vi "ProdaNG.TestStep.Set.vi"(8 "error in (no error)":errorcluster, 9 "ReleaseId":T1=enum."released", 10 "TestStep":T2, 11 "dbHandleIn":i32) -> (0 "error out":errorcluster, 2 "TestStep out":T2, 3 "dbHandle":i32)   [LabVIEW 2016]
doc: "This function returns a product structure for a product, which is identified by a part and a serial number.\nImportant information: The field 'individual' was taken over from the field 'allgemein' of the legacy data directly. Because of this most products have the value 0 further on and only a few the value 1. \nParameter:\nhandle is an Integer, which is returned by the function Login() at the creation of a new connection.\nwabcoPartId is the Id of the part.\nserialNumber is the serial number of the product for the part above.\nproduct is a pointer on a product structure, which is filled if the returncode is 0. The structure must be defined in the calling program.\n\nReturncodes:\n0 No error\n< 0 ORACLE Error code\n6 (ERROR_INVALID_HANDLE) in case of an invalid handle\n1403 Record does not exist"
uses:
  Controls/ProdaNG.TestStep.ctl
  Controls/ProdaNG.ReleaseId.ctl
  Controls/ProdaNG.TestStepSize.ctl
  prodllNG.dll
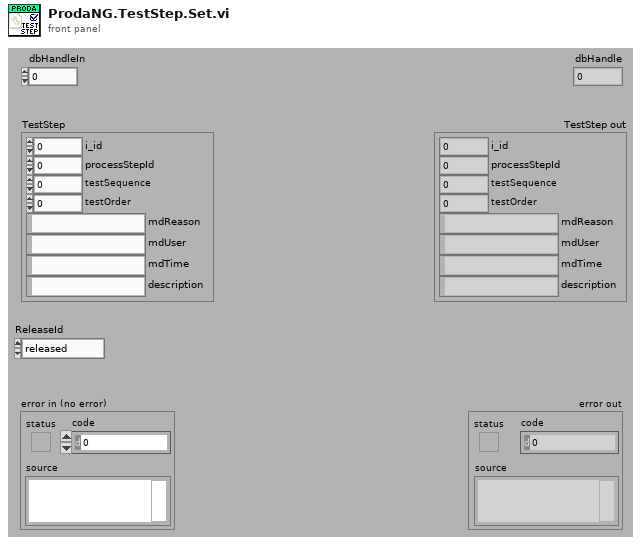
[diagram p1: front panel]
types:
  T1 = typedef "ProdaNG.ReleaseId.ctl" = enum16{"not released", "released", "was released"}
  T2 = typedef "ProdaNG.TestStep.ctl" = cluster{"i_id":i32, "processStepId":i32, "testSequence":i32, "testOrder":i32, "mdReason":string, "mdUser":string, "mdTime":string, "description":string}
  T3 = typedef "ProdaNG.TestStepSize.ctl" = cluster{"i_id":i32, "processStepId":i32, "testSequence":i32, "testOrder":i32, "mdReason":i32, "mdUser":i32, "mdTime":i32, "description":i32}
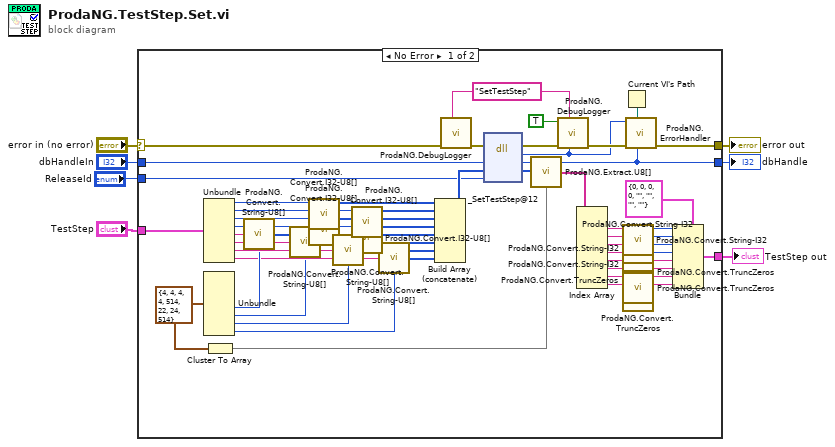
[diagram p0: block diagram]
diagram:
  n1 = case shown="No Error" "error in (no error)" {
    selector: "error in (no error)" -> [w58 w65]
    tunnel: [w63 w65] -> w6
    tunnel: "dbHandleIn" -> [w60 w64]
    tunnel: [w61 w64] -> w4
    tunnel: "TestStep" -> [w24 _]
    tunnel: [w9 _] -> w2
    tunnel: "ReleaseId" -> [w8 _]
    frame No Error {
      w25 = T3 {"i_id"=4, "processStepId"=4, "testSequence"=4, "testOrder"=4, "mdReason"=514, "mdUser"=22, "mdTime"=24, "description"=514} ("TestStepSize")
      w54 = "SetTestStep" ("cmd")
      n2 = Unbundle(w24) -> ("i_id"=w50:i32, "processStepId"=w51:i32, "testSequence"=w20:i32, "testOrder"=w19:i32, "mdReason"=w48:string, "mdUser"=w16:string, "mdTime"=w46:string, "description"=w15:string)
      n3 = Unbundle(w25) -> ("mdReason"=w44:i32, "mdUser"=w12:i32, "mdTime"=w43:i32, "description"=w13:i32)  [unwired: 4 out]
      n4 = Cluster To Array(cluster=w25) -> (array=w21:i32[])
      n5 = call "ProdaNG.Convert.String-U8[].vi"("Input String"=w48, "Size"=w44) -> ("Output"=w47:u8[])
      n6 = call "ProdaNG.Convert.String-U8[].vi"("Input String"=w16, "Size"=w12) -> ("Output"=w10:u8[])
      n7 = call "ProdaNG.Convert.I32-U8[].vi"("32bit integer"=w50) -> ("unsigned byte array"=w49:u8[])  [unwired: 10 in]
      n8 = call "ProdaNG.Convert.I32-U8[].vi"("32bit integer"=w20) -> ("unsigned byte array"=w17:u8[])  [unwired: 10 in]
      n9 = call "ProdaNG.Convert.String-U8[].vi"("Input String"=w46, "Size"=w43) -> ("Output"=w45:u8[])
      n10 = call "ProdaNG.Convert.I32-U8[].vi"("32bit integer"=w51) -> ("unsigned byte array"=w52:u8[])  [unwired: 10 in]
      n11 = call "ProdaNG.Convert.I32-U8[].vi"("32bit integer"=w19) -> ("unsigned byte array"=w18:u8[])  [unwired: 10 in]
      n12 = call "ProdaNG.Convert.String-U8[].vi"("Input String"=w15, "Size"=w13) -> ("Output"=w14:u8[])
      n13 = Build Array (concatenate)(w49, w52, w17, w18, w47, w10, w45, w14) -> (w23:u8[])
      n14 = call "ProdaNG.DebugLogger.vi"("cmd"=w54, "error in (no error)"=w58) -> ("error out"=w57:errorcluster)  [unwired: 9 in]
      n15 = dll-call lib="D:/Maszup/WABCO/SVN/LineTraceSystem/SOFTWARE/sources/Database/ProdaNG/prodllNG.dll" fn="_SetTestStep@12" ("ProDLL wrapper.dll:ProDLL_wrapper_GetWabcoParts_GetData")(error in=w57, "dbHandle"=w60, "testStep"=w23, "releaseId"=w8) -> (error out=w56:errorcluster, "return type"=w53:i32, "dbHandle"=w61:i32, "testStep"=w22:u8[])  [unwired: 3 in, 1 out]
      n16 = call "ProdaNG.Extract.U8[].vi"("unsigned byte array"=w22, "Sizes"=w21) -> ("Elements"=w42:string[])
      n17 = call "ProdaNG.DebugLogger.vi"("return type"=w53, "cmd"=w54, "error in (no error)"=w56, "done? (F)"=TRUE) -> ("error out"=w55:errorcluster)  [unwired: 7 in]
      n18 = Index Array(array=w42) -> (element #1=w41:string, element #2=w38:string, element #3=w37:string, element #4=w31:string, element #5=w28:string, element #6=w27:string, element #7=w32:string, element #8=w34:string)  [unwired: 8 in]
      n19 = Current VI's Path() -> (path=w62:path)
      n20 = call "ProdaNG.Convert.String-I32.vi"("unsigned byte string"=w41) -> ("32bit integer"=w40:i32)  [unwired: 10 in]
      n21 = call "ProdaNG.Convert.String-I32.vi"("unsigned byte string"=w38) -> ("32bit integer"=w39:i32)  [unwired: 10 in]
      n22 = call "ProdaNG.Convert.String-I32.vi"("unsigned byte string"=w37) -> ("32bit integer"=w36:i32)  [unwired: 10 in]
      n23 = call "ProdaNG.Convert.String-I32.vi"("unsigned byte string"=w31) -> ("32bit integer"=w30:i32)  [unwired: 10 in]
      n24 = call "ProdaNG.Convert.TruncZeros.vi"("string with \\0s"=w28) -> ("LV string"=w29:string)  [unwired: 10 in]
      n25 = call "ProdaNG.Convert.TruncZeros.vi"("string with \\0s"=w27) -> ("LV string"=w26:string)  [unwired: 10 in]
      n26 = call "ProdaNG.Convert.TruncZeros.vi"("string with \\0s"=w32) -> ("LV string"=w33:string)  [unwired: 10 in]
      n27 = call "ProdaNG.Convert.TruncZeros.vi"("string with \\0s"=w34) -> ("LV string"=w35:string)  [unwired: 10 in]
      n28 = call "ProdaNG.ErrorHandler.vi"("dbHandleIn"=w61, "Path"=w62, "error in"=w55, "output_parameter"=w53) -> ("error out"=w63:errorcluster)  [unwired: 7 in]
      n29 = Bundle(cluster=T2 {"i_id"=0, "processStepId"=0, "testSequence"=0, "testOrder"=0, "mdReason"="", "mdUser"="", "mdTime"="", "description"=""} ("TestStep"), "i_id"=w40, "processStepId"=w39, "testSequence"=w36, "testOrder"=w30, "mdReason"=w29, "mdUser"=w26, "mdTime"=w33, "description"=w35) -> (w9:T2)
    }
    frame Error {
    }
  }
  "error out" <- w6
  "dbHandle" <- w4
  "TestStep out" <- w2
